vi "Stop Core.vi"(10 "final error code":i32, 11 "MonitoredMediator in":refnum<class "MonitoredMediator.lvclass">) -> (3 "MonitoredMediator out":refnum<class "MonitoredMediator.lvclass">)   [LabVIEW 2019, in "MonitoredMediator.lvlib" / "MonitoredMediator.lvclass"]
doc: "(<B>Filename</B>: Actor Framework.lvlib:Actor.lvclass:Stop Core.vi)\n\nDefines what the actor does before it stops. Use the <B>final error code</B> input to determine whether the actor shut down in response to an error.\n\nBy default, this method does nothing. A descendant class may override it to define behavior, such as shutting down any processes the actor initiated in its override of the Actor Core method."
uses:
  <vilib>/gpm_packages/@cs/mva-core/Source/MonitoredMediator/MonitoredMediator/MonitoredMediator.lvclass
  <vilib>/gpm_packages/@cs/mva-core/Source/MonitoredMediator/MonitoredMediator/MonitoredMediator.lvclass/MonitoredMediator.ctl
  <vilib>/gpm_packages/@cs/mva-core/Source/Mediator/Mediator/Mediator.lvclass
  <vilib>/gpm_packages/@cs/mva-core/Source/MonitoredMediator/IBusMonitor/IBusMonitor.lvclass
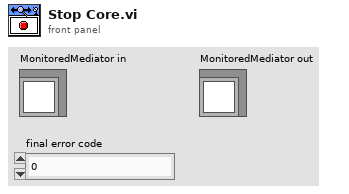
[diagram p1: front panel]
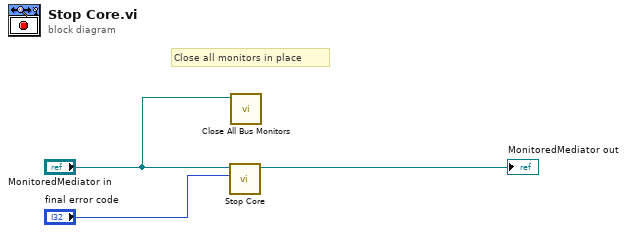
[diagram p0: block diagram]
diagram:
  # "Close all monitors in place"
  n1 = call-parent "Stop Core.vi"("final error code"="final error code", "Mediator in"="MonitoredMediator in") -> ("Mediator out"=→"MonitoredMediator out":refnum<class "MonitoredMediator.lvclass">)  [unwired: 9 in]
  n2 = call <vilib>:"Close All Bus Monitors.vi"("MonitoredMediator in"="MonitoredMediator in") -> ()  [unwired: 10 in, 1 out]
